vi "TrajectoryREADARRAYBEGIN.vi"(10 "Trajectories Files":string[](array[string]), 11 "Trajectory Number 0-x":i32) -> (2 "Trajectory Items":i32, 3 "TotalTImeSecs":dbl)   [LabVIEW 2020]
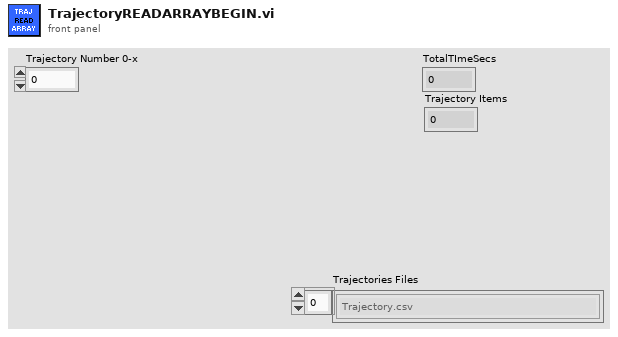
[diagram p1: front panel]
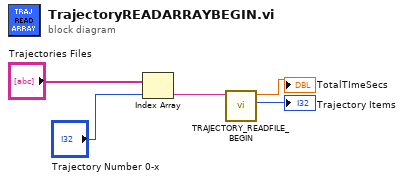
[diagram p0: block diagram]
diagram:
  n1 = Index Array(array="Trajectories Files", index="Trajectory Number 0-x") -> (element=w1:string)
  n2 = call "TRAJECTORY_READFILE_BEGIN.vi"("Trajectory File Name"=w1) -> ("Trajectory Items"=→"Trajectory Items":i32, "TotalTImeSecs"=→"TotalTImeSecs":dbl)  [unwired: 8 in, 1 out]
